vi "Serialize - JSON.vi"(8 "error in":errorcluster, 11 "CRDS Cell Data in":refnum<class "CRDS Cell Data.lvclass">) -> (0 "error out":errorcluster, 2 "Serialized JSON":string, 3 "CRDS Cell Data out":refnum<class "CRDS Cell Data.lvclass">)   [LabVIEW 2014, in "CRDS Lib.lvlib" / "CRDS Cell Data.lvclass"]
uses:
  CRDS Cell Data.lvclass
  Cell/extParam Ctl.ctl
  Cell/hkParam Ctl.ctl
  CRDS Cell Data.lvclass/CRDS Cell Data.ctl
  CRDS Lib.lvlib
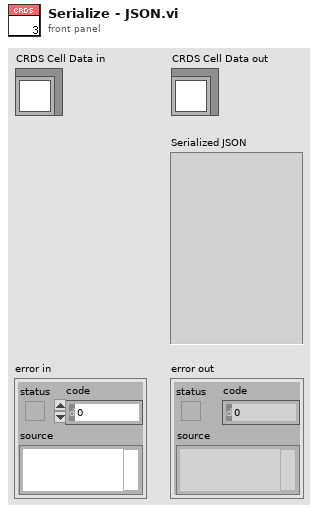
[diagram p1: front panel]
types:
  T1 = typedef "CRDS Lib.lvlib/extParam Ctl.ctl" = cluster{"Tau":sgl, "Tau0cor":sgl, "ext":sgl, "extCorr":sgl, "stdevTau":sgl, "eTau":sgl, "taucorr":sgl, "Tau0":sgl, "max":sgl}
  T2 = typedef "hkParam Ctl.ctl" = cluster{"rhDilFac":sgl, "Q":sgl, "Tmean":sgl, "extDilFac":sgl, "rhCell":sgl, "P":sgl, "T":sgl}
  T3 = cluster{"extParam":T1, "hkData":T2, "Ringdowns":i16[][]}
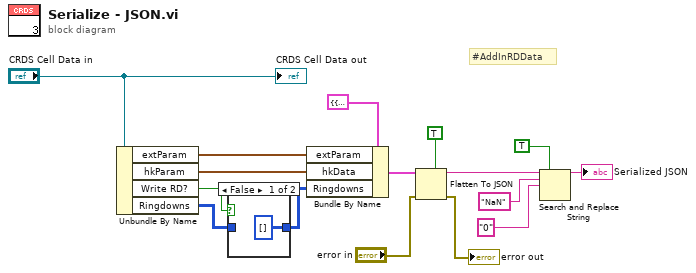
[diagram p0: block diagram]
diagram:
  # "#AddInRDData"
  n1 = Unbundle By Name("CRDS Cell Data in") -> ("extParam"=w14:T1, "hkParam"=w13:T2, "Write RD?"=w5:bool, "Ringdowns"=w4:i16[][])
  n2 = case shown="False" w5 {
    tunnel: w4 -> [_ w18]
    tunnel: [i16[][] [] ("Ringdowns") w18] -> w3
    frame False {
    }
    frame True {
    }
  }
  n3 = Bundle By Name(cluster=T3 {"extParam"={"Tau"=0.0, "Tau0cor"=0.0, "ext"=0.0, "extCorr"=0.0, "stdevTau"=0.0, "eTau"=0.0, "taucorr"=0.0, "Tau0"=0.0, "max"=0.0}, "hkData"={"rhDilFac"=0.0, "Q"=0.0, "Tmean"=0.0, "extDilFac"=0.0, "rhCell"=0.0, "P"=0.0, "T"=0.0}, "Ringdowns"=[]} ("CellData"), "extParam"=w14, "hkData"=w13, "Ringdowns"=w3) -> (w12:T3)
  n4 = Flatten To JSON(enable LabVIEW extensions? (T)=TRUE, anything=w12, error in (no error)="error in") -> (JSON string=w10:string, 11:→"error out":errorcluster)
  n5 = Search and Replace String(replace all?=TRUE ("replace all? (F)"), input string=w10, search string="NaN", replace string="0" ("replace string (\"\")")) -> (result string=→"Serialized JSON":string)  [unwired: 4 in, 3 out]
  "CRDS Cell Data out" <- "CRDS Cell Data in"
